vi "ECS-1408-FPGA1-EPTx.vi"() -> ()   [LabVIEW 2015, in "ECS-FPGA.lvlib"]
uses:
  ECS-FPGA.lvlib
  <vilib>/Powertrain Controls/Device Drivers/Engine Position Tracking/EPTx/RevA/FPGA/Controls/EPTxSupervisor.ctl
  <vilib>/Powertrain Controls/Device Drivers/Engine Position Tracking/EPTx/RevA/FPGA/Controls/EPTxConfig.ctl
  <vilib>/Powertrain Controls/Device Drivers/Engine Position Tracking/EPTx/RevA/FPGA/Controls/EPTxControl.ctl
  <vilib>/Powertrain Controls/Device Drivers/Engine Position Tracking/EPTx/RevA/FPGA/Controls/EPTxTooth.ctl
  <vilib>/Powertrain Controls/Device Drivers/Engine Position Tracking/EPTx/RevA/FPGA/Controls/EPTxAAPControl.ctl
  <vilib>/Powertrain Controls/Device Drivers/Engine Position Tracking/EPTx/RevA/FPGA/Controls/EPTxFuelSparkControl.ctl
  <vilib>/Platform/TimedLoop/XDataNode/timing_clust.ctl
  <vilib>/Platform/TimedLoop/XDataNode/nitl_modes.ctl
  <vilib>/Platform/TimedLoop/XDataNode/wakeup.ctl
  <vilib>/Powertrain Controls/Device Drivers/Engine Position Tracking/EPTx/RevA/FPGA/Controls/EPTxSignals.ctl
  <vilib>/rvi/Emulation/niFpgaSctlEmulationGetInTimedLoop.vi
  <vilib>/rvi/Emulation/niFpgaEmulationReportErrorSimple.vi
  <vilib>/rvi/Emulation/niFpgaGetClockAttributes.vi
  <vilib>/rvi/Emulation/niFpgaCriticalErrorInLSC.vi
  <vilib>/rvi/eio/common/nirviEmuTemplateMethod_errors.vi
  <vilib>/Platform/TimedLoop/XDataNode/XDataNode.xnode
  <vilib>/eio/EIONode/EIONode.xnode
  <vilib>/Platform/TimedLoop/XDataNode/XDNodeRunTimeDep.lvlib
  <vilib>/Powertrain Controls/Device Drivers/Engine Position Tracking/EPTx/RevA/FPGA/EPTx - RevA - FPGA.lvlib
panel:
  in  "O2-1.Control":T1
  out "O2-1.Data":T2
  in  "DI-1.PlsGen_Config_Channel3":T3
  in  "DI-1.PlsGen_Config_Channel2":T3
  in  "DI-1.PlsGen_Config_Channel1":T3
  in  "PFI-1.FuelControl 4":T4
  in  "PFI-1.FuelControl 3":T4
  in  "PFI-1.FuelControl 2":T4
  in  "PFI-1.FuelControl 1":T4
  out "EPTx.Aux4CaptureCAD":fxp<+,18,11>
  out "EPTx.Aux3CaptureCAD":fxp<+,18,11>
  out "EPTx.Aux2CaptureCAD":fxp<+,18,11>
  out "EPTx.Aux1CaptureCAD":fxp<+,18,11>
  out "EPTx.Aux4EdgeCount":u8
  out "EPTx.Aux3EdgeCount":u8
  out "EPTx.Aux2EdgeCount":u8
  out "EPTx.Aux1EdgeCount":u8
  in  "EPTx.Aux4AngleCapture":T5
  in  "EPTx.Aux3AngleCapture":T5
  in  "EPTx.Aux2AngleCapture":T5
  in  "EPTx.Aux1AngleCapture":T5
  out "EPTxTooth":T6
  in  "EPTxControl":T7
  in  "EPTxConfig":T8
  out "EPTxSupervisor":T9
  out "ADCombo-1.DigitalTriggers":u32
  out "Throttle-1.Data":T10 caption="ThrottleData"
  in  "Throttle-1.Control":T11 caption="ThrottleControl"
  out "ADCombo-1.VRHallData":T12 caption="VRHallData"
  in  "EPTx.Aux4":u8=2
  in  "EPTx.Aux2":u8=1
  out "DI-1.Data":T13 caption="DIData"
  in  "ADCombo-1.VRHallInvert":u8
  in  "ADCombo-1.VR1.Filt":u16
  in  "ADCombo-1.VR2.Filt":u16
  in  "ADCombo-1.Hall1.Filt":u16
  in  "ADCombo-1.Hall2.Filt":u16
  in  "9411-1.0.Filt":u16
  in  "9411-1.1.Filt":u16
  in  "9411-1.2.Filt":u16
  in  "9411-1.3.Filt":u16
  in  "9411-1.4.Filt":u16
  in  "9411-1.5.Filt":u16
  in  "9411-1.Invert":u8
  out "ADCombo-1.ModulePresent":bool caption="ModulePresent"
  out "PFI-1.Data":T14 caption="PFIData"
  in  "PFI-1.IPhaseInterface":T15(array[cluster])=[{"IPhaseCurrent"=0, "IPhaseDuration"=0}, {"IPhaseCurrent"=0, "IPhaseDuration"=0}, {"IPhaseCurrent"=0, "IPhaseDuration"=0}, {"IPhaseCurrent"=0, "IPhaseDuration"=0}, {"IPhaseCurrent"=0, "IPhaseDuration"=0}, {"IPhaseCurrent"=0, "IPhaseDuration"=0}, {"IPhaseCurrent"=0, "IPhaseDuration"=0}, {"IPhaseCurrent"=0, "IPhaseDuration"=0}] caption="IPhaseInterface"
  in  "PFI-1.LowsidePWM":T16 caption="LowsidePWM"
  in  "PFI-1.Control":T17 caption="PFIControl"
  out "DI-1.ScopeData":T18 caption="DIScopeData"
  in  "DI-1.ScopeRead":bool caption="DIScopeRead"
  in  "DI-1.IPhaseInterface":T19(array[cluster]) caption="IPhaseInterface"
  in  "DI-1.Control":T20 caption="DIControl"
  in  "EPTx.Aux3":u8
  in  "EPTx.Primary":u8
  in  "EPTx.Aux1":u8
  out "ADCombo-1.Hall1.PPWData":T21
  out "ADCombo-1.Hall2.PPWData":T21
  out "ADCombo-1.VR2.PPWData":T21
  out "ADCombo-1.VR1.PPWData":T21
  out "9411-1.0.PPWData":T21
  out "9411-1.1.PPWData":T21
  out "9411-1.2.PPWData":T21
  out "9411-1.3.PPWData":T21
  out "9411-1.4.PPWData":T21
  out "9411-1.5.PPWData":T21
  out "9411-1.DigitalTriggers":u32
  out "ADCombo-1.AnalogData":T22 caption="AnalogData"
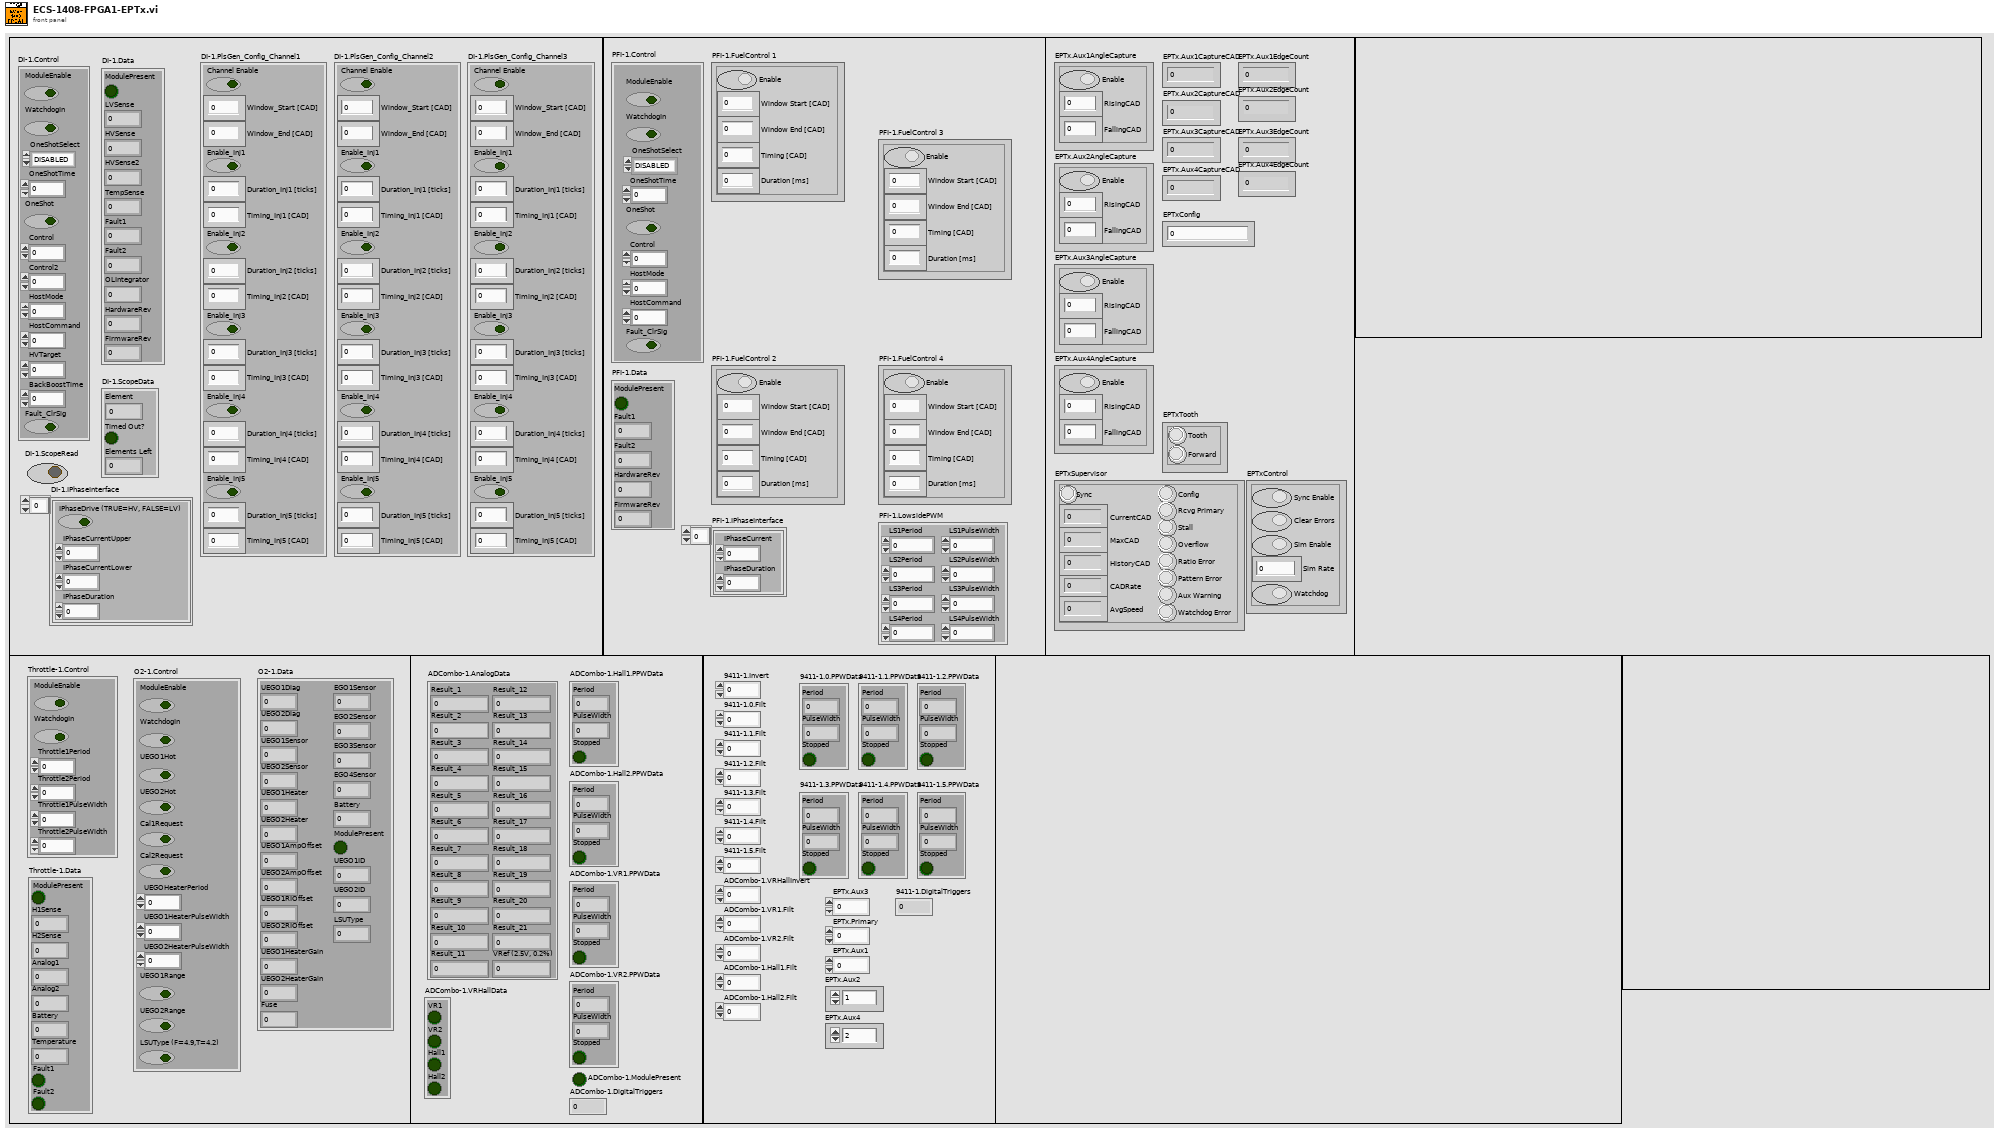
[diagram p1: front panel]
types:
  T1 = cluster{"ModuleEnable":bool, "WatchdogIn":bool, "UEGO1Hot":bool, "UEGO2Hot":bool, "Cal1Request":bool, "Cal2Request":bool, "UEGOHeaterPeriod":u16, "UEGO1HeaterPulseWidth":u16, "UEGO2HeaterPulseWidth":u16, "UEGO1Range":bool, "UEGO2Range":bool, "LSUType (F=4.9,T=4.2)":bool}
  T2 = cluster{"UEGO1Diag":u8, "UEGO2Diag":u8, "UEGO1Sensor":u16, "UEGO2Sensor":u16, "UEGO1Heater":u16, "UEGO2Heater":u16, "UEGO1AmpOffset":u16, "UEGO2AmpOffset":u16, "UEGO1RIOffset":u16, "UEGO2RIOffset":u16, "UEGO1HeaterGain":u16, "UEGO2HeaterGain":u16, "Fuse":u16, "EGO1Sensor":u16, "EGO2Sensor":u16, "EGO3Sensor":u16, "EGO4Sensor":u16, "Battery":u16, "ModulePresent":bool, "UEGO1ID":u8, "UEGO2ID":u8, "LSUType":u8}
  T3 = cluster{"Channel Enable":bool, "Window_Start [CAD]":fxp<+,18,11>, "Window_End [CAD]":fxp<+,18,11>, "Enable_Inj1":bool, "Duration_Inj1 [ticks]":u32, "Timing_Inj1 [CAD]":fxp<+,18,11>, "Enable_Inj2":bool, "Duration_Inj2 [ticks]":u32, "Timing_Inj2 [CAD]":fxp<+,18,11>, "Enable_Inj3":bool, "Duration_Inj3 [ticks]":u32, "Timing_Inj3 [CAD]":fxp<+,18,11>, "Enable_Inj4":bool, "Duration_Inj4 [ticks]":u32, "Timing_Inj4 [CAD]":fxp<+,18,11>, "Enable_Inj5":bool, "Duration_Inj5 [ticks]":u32, "Timing_Inj5 [CAD]":fxp<+,18,11>}
  T4 = typedef "EPTx - RevA - FPGA.lvlib/EPTxFuelSparkControl.ctl" = cluster{"Enable":bool, "Window Start [CAD]":fxp<+,18,11>, "Window End [CAD]":fxp<+,18,11>, "Timing [CAD]":fxp<+,18,11>, "Duration [ms]":fxp<+/-,22,9>}
  T5 = typedef "EPTx - RevA - FPGA.lvlib/EPTxAAPControl.ctl" = cluster{"Enable":bool, "RisingCAD":fxp<+,18,11>, "FallingCAD":fxp<+,18,11>}
  T6 = typedef "EPTx - RevA - FPGA.lvlib/EPTxTooth.ctl" = cluster{"Tooth":bool, "Forward":bool}
  T7 = typedef "EPTx - RevA - FPGA.lvlib/EPTxControl.ctl" = cluster{"Sync Enable":bool, "Clear Errors":bool, "Sim Enable":bool, "Sim Rate":fxp<+,24,6>, "Watchdog":bool}
  T8 = typedef "EPTx - RevA - FPGA.lvlib/EPTxConfig.ctl" = u64
  T9 = typedef "EPTx - RevA - FPGA.lvlib/EPTxSupervisor.ctl" = cluster{"Sync":bool, "CurrentCAD":fxp<+,18,11>, "MaxCAD":fxp<+,11,11>, "HistoryCAD":fxp<+,11,11>, "CADRate":fxp<+,22,8>, "AvgSpeed":fxp<+,17,15>, "Config":bool, "Rcvg Primary":bool, "Stall":bool, "Overflow":bool, "Ratio Error":bool, "Pattern Error":bool, "Aux Warning":bool, "Watchdog Error":bool}
  T10 = cluster{"ModulePresent":bool, "H1Sense":i16, "H2Sense":i16, "Analog1":i16, "Analog2":i16, "Battery":i16, "Temperature":i16, "Fault1":bool, "Fault2":bool}
  T11 = cluster{"ModuleEnable":bool, "WatchdogIn":bool, "Throttle1Period":u16, "Throttle2Period":u16, "Throttle1PulseWidth":i16, "Throttle2PulseWidth":i16}
  T12 = cluster{"VR1":bool, "VR2":bool, "Hall1":bool, "Hall2":bool}
  T13 = cluster{"ModulePresent":bool, "LVSense":u8, "HVSense":u8, "HVSense2":u8, "TempSense":i8, "Fault1":u8, "Fault2":u8, "OLIntegrator":u32, "HardwareRev":u8, "FirmwareRev":u8}
  T14 = cluster{"ModulePresent":bool, "Fault1":u8, "Fault2":u8, "HardwareRev":u8, "FirmwareRev":u8}
  T15 = cluster{"IPhaseCurrent":u16, "IPhaseDuration":u16}[]
  T16 = cluster{"LS1Period":u32, "LS1PulseWidth":u32, "LS2Period":u32, "LS2PulseWidth":u32, "LS3Period":u32, "LS3PulseWidth":u32, "LS4Period":u32, "LS4PulseWidth":u32}
  T17 = cluster{"ModuleEnable":bool, "WatchdogIn":bool, "OneShotSelect":enum8{"DISABLED", "PFI 1", "PFI 2", "PFI 3", "PFI 4"}, "OneShotTime":u32, "OneShot":bool, "Control":u16, "HostMode":u8, "HostCommand":u32, "Fault_ClrSig":bool}
  T18 = cluster{"Element":u32, "Timed Out?":bool, "Elements Left":u32}
  T19 = cluster{"IPhaseDrive (TRUE=HV, FALSE=LV)":bool, "IPhaseCurrentUpper":u16, "IPhaseCurrentLower":u16, "IPhaseDuration":u16}[]
  T20 = cluster{"ModuleEnable":bool, "WatchdogIn":bool, "OneShotSelect":enum8{"DISABLED", "CHAN 1", "CHAN 2", "CHAN 3"}, "OneShotTime":u32, "OneShot":bool, "Control":u8, "Control2":u8, "HostMode":u8, "HostCommand":u32, "HVTarget":u8, "BackBoostTime":u8, "Fault_ClrSig":bool}
  T21 = cluster{"Period":u32, "PulseWidth":u32, "Stopped":bool}
  T22 = cluster{"Result_1":u16, "Result_2":u16, "Result_3":u16, "Result_4":u16, "Result_5":u16, "Result_6":u16, "Result_7":u16, "Result_8":u16, "Result_9":u16, "Result_10":u16, "Result_11":u16, "Result_12":u16, "Result_13":u16, "Result_14":u16, "Result_15":u16, "Result_16":u16, "Result_17":u16, "Result_18":u16, "Result_19":u16, "Result_20":u16, "Result_21":u16, "VRef (2.5V, 0.2%)":u16}
  T23 = typedef "XDNodeRunTimeDep.lvlib/timing_clust.ctl" = cluster{"Expected End [f-1]":u64, "Actual End [f-1]":u64, "Finished Late? [f-1]":bool, "Expected End [i-1]":u64, "Actual End [i-1]":u64, "Finished Late? [i-1]":bool, "Expected Start [i]":u64, "Actual Start [i]":u64, "Expected Start [f]":u64, "Actual Start [f]":u64, "Source Name":string, "Structure Name":string, "Period":i64, "Deadline":i64, "Offset":i64, "Start":i64, "Priority":i32, "Timeout":i32, "Mode":T24, "Wakeup Reason":T25, "Error":errorcluster, "Source Type":string, "Secondary Source Type":string, "Global End Time":u64, "Global Start Time":u64, "Frame Duration":u64, "Iteration Duration":u64, "Assigned CPU":i32, "I/O Scan Engine Mode":u32}
  T24 = typedef "XDNodeRunTimeDep.lvlib/nitl_modes.ctl" = enum32{"No Change", "Process missed periods, maintain original phase", "Discard missed periods, maintain original phase", "Process missed periods, ignore original phase", "Discard missed periods, ignore original phase"}
  T25 = typedef "XDNodeRunTimeDep.lvlib/wakeup.ctl" = enum32{"Normal", "Aborted", "Asynchronous wakeup", "Timing source error", "Timed loop error", "Timeout"}
  T26 = typedef "EPTx - RevA - FPGA.lvlib/EPTxSignals.ctl" = cluster{"Primary":bool, "Aux 1":bool, "Aux 2":bool, "Aux 3":bool, "Aux 4":bool}
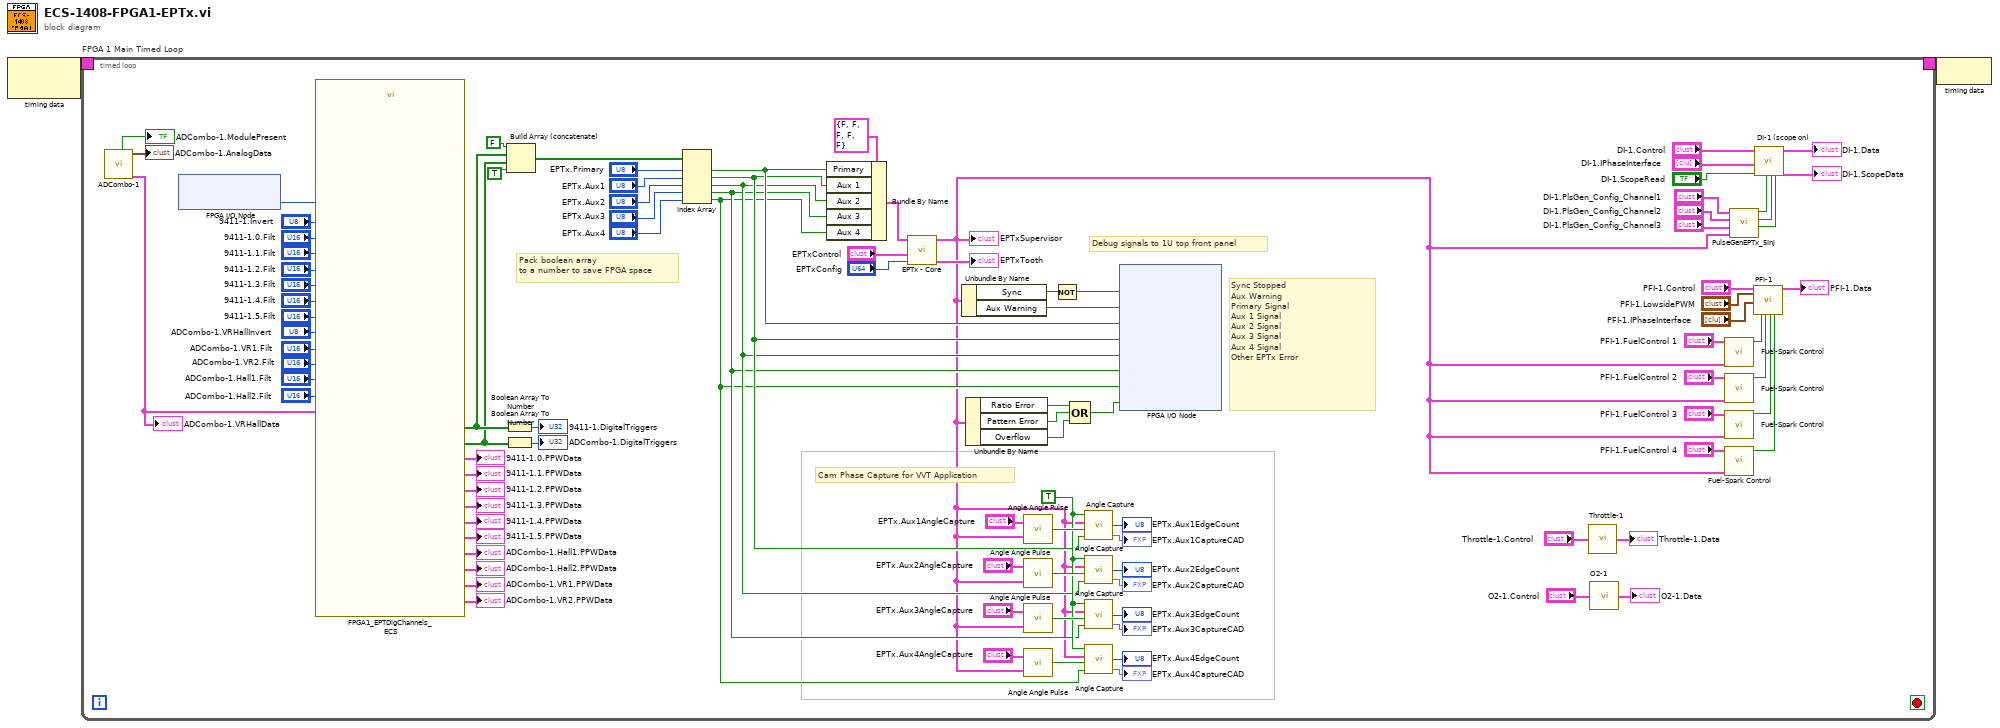
[diagram p0: block diagram]
diagram:
  n1 = node-c288() -> (w2:T23)  [unwired: 1 in]
  n2 = timed-loop "FPGA 1 Main Timed Loop" {
    timing: w2 -> [_]
    timing-out: [_] -> w1
    stop <- _ stop-if-true
    w39 = TRUE ("Enable")
    # "Pack boolean array\nto a number to save FPGA space"
    # "Cam Phase Capture for VVT Application"
    # "Debug signals to 1U top front panel"
    # "Sync Stopped\nAux Warning\nPrimary Signal\nAux 1 Signal\nAux 2 Signal\nAux 3 Signal\nAux 4 Signal\nOther EPTx Error"
    n3 = call "ADCombo-1"() -> ("ADCombo-1_VRHallData"=w102:T12, "ADCombo-1_AnalogData"=→"ADCombo-1.AnalogData":T22, "ADCombo-1_ModulePresent"=→"ADCombo-1.ModulePresent":bool)  [unwired: 5 in, 2 out]
    "ADCombo-1.VRHallData" <- w102
    n4 = xnode "FPGA I/O Node"() -> ("9411-1/DI5:0"=w99:u8)  [unwired: 1 in, 1 out]
    n5 = call "FPGA1_EPTDigChannels_ECS.vi"("NI9411-1.2.Filt"="9411-1.2.Filt", "NI9411-1.3.Filt"="9411-1.3.Filt", "NI9411-1.4.Filt"="9411-1.4.Filt", "NI9411-1.5.Filt"="9411-1.5.Filt", "ADCombo-1.VRHallData"=w102, "ADCombo-1.VR1.Filt"="ADCombo-1.VR1.Filt", "ADCombo-1.VR2.Filt"="ADCombo-1.VR2.Filt", "9411/DI5:0"=w99, "ADCombo-1.Hall1.Filt"="ADCombo-1.Hall1.Filt", "NI9411-1.1.Filt"="9411-1.1.Filt", "ADCombo-1.Hall2.Filt"="ADCombo-1.Hall2.Filt", "NI9411-1.Invert"="9411-1.Invert", "ADCombo-1.VRHallInvert"="ADCombo-1.VRHallInvert", "NI9411-1.0.Filt"="9411-1.0.Filt") -> ("9411-1.0.PPWData"=→"9411-1.0.PPWData":T21, "ADCombo-1.Hall2.PPWData"=→"ADCombo-1.Hall2.PPWData":T21, "9411-1.1.PPWData"=→"9411-1.1.PPWData":T21, "ADCombo-1.Hall1.PPWData"=→"ADCombo-1.Hall1.PPWData":T21, "9411-1.2.PPWData"=→"9411-1.2.PPWData":T21, "9411-1.3.PPWData"=→"9411-1.3.PPWData":T21, "9411-1.4.PPWData"=→"9411-1.4.PPWData":T21, "9411-1.5.PPWData"=→"9411-1.5.PPWData":T21, "9411-1.DigitalTriggers"=w58:bool[], "ADCombo-1.VR1.PPWData"=→"ADCombo-1.VR1.PPWData":T21, "ADCombo-1.VR2.PPWData"=→"ADCombo-1.VR2.PPWData":T21, "ADCombo-1.DigitalTriggers"=w57:bool[])  [unwired: 2 in]
    n6 = Boolean Array To Number(Boolean array=w58) -> (number=→"9411-1.DigitalTriggers":u32)
    n7 = Boolean Array To Number(Boolean array=w57) -> (number=→"ADCombo-1.DigitalTriggers":u32)
    n8 = Build Array (concatenate)(FALSE, w58, w57, TRUE) -> (w48:bool[])
    n9 = Index Array(array=w48, index #1="EPTx.Primary", index #2="EPTx.Aux1", index #3="EPTx.Aux2", index #4="EPTx.Aux3", index #5="EPTx.Aux4") -> (element #1=w20:bool, element #2=w19:bool, element #3=w18:bool, element #4=w17:bool, element #5=w16:bool)
    n10 = Bundle By Name(cluster=T26 {"Primary"=FALSE, "Aux 1"=FALSE, "Aux 2"=FALSE, "Aux 3"=FALSE, "Aux 4"=FALSE} ("EPTxSignals"), "Primary"=w20, "Aux 1"=w19, "Aux 2"=w18, "Aux 3"=w17, "Aux 4"=w16) -> (w51:T26)
    n11 = call <vilib>:"EPTx - Core.vi"("EPTxConfig"="EPTxConfig", "EPTxControl"="EPTxControl", "EPTxSignals"=w51) -> ("EPTxTooth"=→"EPTxTooth":T6, "EPTxSupervisor"=w8:T9)  [unwired: 7 in]
    "EPTxSupervisor" <- w8
    n12 = Unbundle By Name(w8) -> ("Sync"=w49:bool, "Aux Warning"=w21:bool)
    n13 = Unbundle By Name(w8) -> ("Ratio Error"=w15:bool, "Pattern Error"=w14:bool, "Overflow"=w13:bool)
    n14 = call <vilib>:"Angle Angle Pulse.vi"("EPTxSupervisor"=w8, "AAPControl"="EPTx.Aux1AngleCapture") -> ("AAP"=w45:bool)
    n15 = call <vilib>:"Angle Angle Pulse.vi"("EPTxSupervisor"=w8, "AAPControl"="EPTx.Aux2AngleCapture") -> ("AAP"=w44:bool)
    n16 = call <vilib>:"Angle Angle Pulse.vi"("EPTxSupervisor"=w8, "AAPControl"="EPTx.Aux3AngleCapture") -> ("AAP"=w43:bool)
    n17 = call <vilib>:"Angle Angle Pulse.vi"("EPTxSupervisor"=w8, "AAPControl"="EPTx.Aux4AngleCapture") -> ("AAP"=w40:bool)
    n18 = Not(x=w49) -> (.not. x?=w22:bool)
    n19 = Compound Arithmetic op=OR(w15, w14, w13) -> (w12:bool)
    n20 = call <vilib>:"Angle Capture.vi"("Capture"=w19, "OpWindow"=w45, "EPTxSupervisor"=w8, "Enable"=w39) -> ("CaptureCAD"=→"EPTx.Aux1CaptureCAD":fxp<+,18,11>, "CaptureCount"=→"EPTx.Aux1EdgeCount":u8)  [unwired: 1 out]
    n21 = call <vilib>:"Angle Capture.vi"("Capture"=w18, "OpWindow"=w44, "EPTxSupervisor"=w8, "Enable"=w39) -> ("CaptureCAD"=→"EPTx.Aux2CaptureCAD":fxp<+,18,11>, "CaptureCount"=→"EPTx.Aux2EdgeCount":u8)  [unwired: 1 out]
    n22 = call <vilib>:"Angle Capture.vi"("Capture"=w17, "OpWindow"=w43, "EPTxSupervisor"=w8, "Enable"=w39) -> ("CaptureCAD"=→"EPTx.Aux3CaptureCAD":fxp<+,18,11>, "CaptureCount"=→"EPTx.Aux3EdgeCount":u8)  [unwired: 1 out]
    n23 = call <vilib>:"Angle Capture.vi"("Capture"=w16, "OpWindow"=w40, "EPTxSupervisor"=w8, "Enable"=w39) -> ("CaptureCAD"=→"EPTx.Aux4CaptureCAD":fxp<+,18,11>, "CaptureCount"=→"EPTx.Aux4EdgeCount":u8)  [unwired: 1 out]
    n24 = xnode "FPGA I/O Node"("9401-1/DIO0"=w22, "9401-1/DIO1"=w21, "9401-1/DIO2"=w20, "9401-1/DIO3"=w19, "9401-1/DIO4"=w18, "9401-1/DIO5"=w17, "9401-1/DIO6"=w16, "9401-1/DIO7"=w12) -> ()  [unwired: 8 in, 8 out]
    n25 = call "Throttle-1"("Throttle-1_Control"="Throttle-1.Control") -> ("Throttle-1_Data"=→"Throttle-1.Data":T10)
    n26 = call "O2-1"("O2Control"="O2-1.Control") -> ("O2Data"=→"O2-1.Data":T2)
    n27 = call <vilib>:"Fuel-Spark Control.vi"("EPTxSupervisor"=w8, "Fuel-Spark Control"="PFI-1.FuelControl 1") -> ("Fuel-Spark Command"=w23:bool)  [unwired: 9 in]
    n28 = call <vilib>:"Fuel-Spark Control.vi"("EPTxSupervisor"=w8, "Fuel-Spark Control"="PFI-1.FuelControl 2") -> ("Fuel-Spark Command"=w24:bool)  [unwired: 9 in]
    n29 = call <vilib>:"Fuel-Spark Control.vi"("EPTxSupervisor"=w8, "Fuel-Spark Control"="PFI-1.FuelControl 3") -> ("Fuel-Spark Command"=w25:bool)  [unwired: 9 in]
    n30 = call <vilib>:"Fuel-Spark Control.vi"("EPTxSupervisor"=w8, "Fuel-Spark Control"="PFI-1.FuelControl 4") -> ("Fuel-Spark Command"=w26:bool)  [unwired: 9 in]
    n31 = call "PulseGenEPTx_5Inj.vi"("EPTxSupervisor"=w8, "Inj_Config_Channel3"="DI-1.PlsGen_Config_Channel3", "Inj_Config_Channel2"="DI-1.PlsGen_Config_Channel2", "Inj_Config_Channel1"="DI-1.PlsGen_Config_Channel1") -> ("CmdOut3"=w5:bool, "CmdOut2"=w6:bool, "CmdOut1"=w7:bool)  [unwired: 3 in]
    n32 = call "PFI-1"("PFI-1_Control"="PFI-1.Control", "PFI-1_LowsidePWM"="PFI-1.LowsidePWM", "PFI-1_IPhaseInterface"="PFI-1.IPhaseInterface", "PFI1Cmd"=w23, "PFI2Cmd"=w24, "PFI3Cmd"=w25, "PFI4Cmd"=w26) -> ("PFI-1_Data"=→"PFI-1.Data":T14)  [unwired: 11 in, 1 out]
    n33 = call "DI-1 (scope on)"("DI-1_Control"="DI-1.Control", "DI-1_IPhaseInterface"="DI-1.IPhaseInterface", "DI-1_ScopeRead"="DI-1.ScopeRead", "DI1Cmd"=w7, "DI2Cmd"=w6, "DI3Cmd"=w5) -> ("DI-1_Data"=→"DI-1.Data":T13, "DI-1_ScopeData"=→"DI-1.ScopeData":T18)  [unwired: 11 in, 1 out]
  }
  n34 = node-c288(w1) -> ()
